vi "Read Graph.vi"(8 "error in (no error)":errorcluster, 11 "I-V Result in":refnum<class "I-V Result.lvclass">) -> (0 "error out":errorcluster, 2 "Graph":T1, 3 "I-V Result out":refnum<class "I-V Result.lvclass">)   [LabVIEW 2013, in "Diode Characterization.lvlib" / "I-V Result.lvclass"]
uses:
  I-V Result.lvclass
  graphdata.ctl
  <vilib>/Utility/miscctls.llb/LVAnnotationListTypeDef.ctl
  <vilib>/Utility/miscctls.llb/LVCursorListTypeDef.ctl
  I-V Result.lvclass/I-V Result.ctl
  Diode IV.lvclass
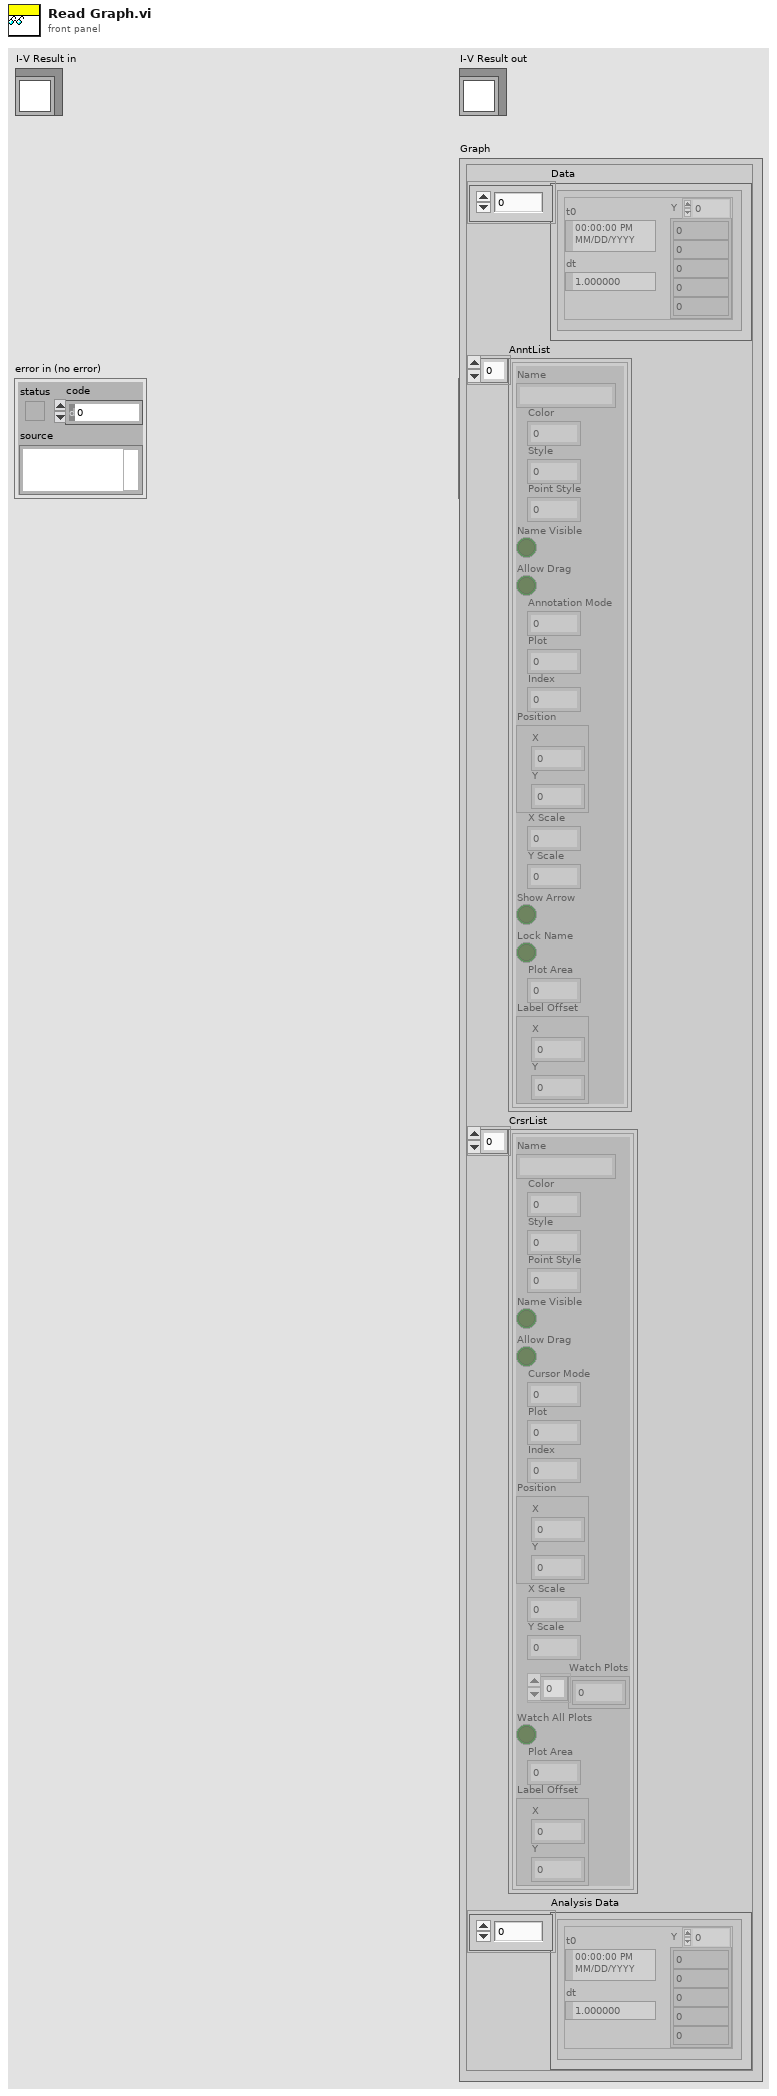
[diagram p1: front panel]
types:
  T1 = typedef "Diode Characterization.lvlib/Diode IV.lvclass/graphdata.ctl" = cluster{"Data":waveform(dbl)[], "AnntList":T2, "CrsrList":T3, "Analysis Data":waveform(dbl)[]}
  T2 = typedef "LVAnnotationListTypeDef.ctl" = cluster{"Name":string, "Color":u32, "Style":u8, "Point Style":u8, "Name Visible":bool, "Allow Drag":bool, "Annotation Mode":u32, "Plot":i32, "Index":i32, "Position":cluster{"X":dbl, "Y":dbl}, "X Scale":u32, "Y Scale":u32, "Show Arrow":bool, "Lock Name":bool, "Plot Area":i32, "Label Offset":cluster{"X":dbl, "Y":dbl}}[]
  T3 = typedef "LVCursorListTypeDef.ctl" = cluster{"Name":string, "Color":u32, "Style":u8, "Point Style":u8, "Name Visible":bool, "Allow Drag":bool, "Cursor Mode":u32, "Plot":i32, "Index":i32, "Position":cluster{"X":dbl, "Y":dbl}, "X Scale":u32, "Y Scale":u32, "Watch Plots":i32[], "Watch All Plots":bool, "Plot Area":i32, "Label Offset":cluster{"X":dbl, "Y":dbl}}[]
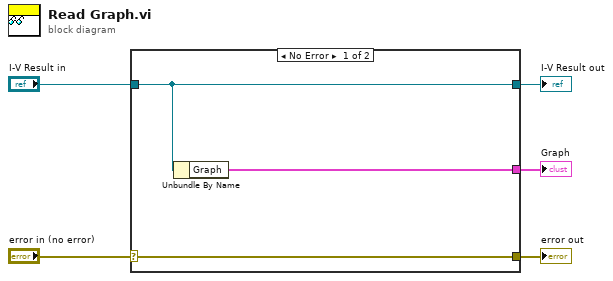
[diagram p0: block diagram]
diagram:
  n1 = case shown="No Error" "error in (no error)" {
    selector: "error in (no error)" -> [w8 w9]
    tunnel: [w8 w9] -> w4
    tunnel: [w7 w10] -> w2
    tunnel: "I-V Result in" -> [w7 w10]
    tunnel: [w6 _] -> w1
    frame No Error {
      n2 = Unbundle By Name(w7) -> ("Graph"=w6:T1)
    }
    frame Error {
    }
  }
  "error out" <- w4
  "I-V Result out" <- w2
  "Graph" <- w1
